vi "Configure Channels.vi"(8 "error in":errorcluster, 11 "DI Cont CFG in":refnum<class "DI DAQmx Cont CFG.lvclass">) -> (0 "error out":errorcluster, 3 "DI Cont CFG out":refnum<class "DI DAQmx Cont CFG.lvclass">)   [LabVIEW 2024, in "DI DAQmx Cont CFG.lvclass"]
uses:
  DI DAQmx Cont CFG.lvclass
  DI DAQmx Cont CFG.lvclass/DI DAQmx Cont CFG.ctl
  DAQmx Base CFG/DAQmx Base CFG.lvclass/DAQmx Base CFG.ctl
  Configurations/CFG Base/CFG Base.lvclass/CFG Base.ctl
  554e4c80-a6e4-4458-875d-47822cf13ff0.vi
  554e4c80-a6e4-4458-875d-47822cf13ff0.vi/a4169a97-72fc-4003-a778-603cf20cafa0.vi
  <vilib>/JDP Science/JSONtext/Find Item.vi
  <vilib>/JDP Science/JSONtext/Next JSON Value.vi
  <vilib>/JDP Science/JSONtext/String Subset.vi
  <vilib>/JDP Science/JSONtext/Parsing/Advance past next JSON Value (inlined COPY).vi
  <vilib>/JDP Science/JSONtext/Parsing/Advance past whitespace.vi
  <vilib>/JDP Science/JSONtext/Parsing/Advance past String.vi
  <vilib>/JDP Science/JSONtext/Parsing/Advance past Number.vi
  <vilib>/JDP Science/JSONtext/Parsing/Advance past Line Ending.vi
  <vilib>/JDP Science/JSONtext/Parsing/Parse Full Path or Item Name.vi
  <vilib>/JDP Science/JSONtext/Parsing/Advance past Array.vi
  <vilib>/JDP Science/JSONtext/Parsing/Advance past Object.vi
  <vilib>/JDP Science/JSONtext/support/Error Cluster From Code.vi
  <vilib>/JDP Science/JSONtext/Offset/Find Item Locations by Path.vi
  <vilib>/JDP Science/JSONtext/JSON text to Variant.vi
  <vilib>/Utility/error.llb/Error Cluster From Error Code.vi
  <vilib>/DAQmx/create/channels.llb/DAQmx Create Channel (DI-Digital Input).vi
  <vilib>/JDP Science/JSONtext/LVClass Serializer/JSONtext LVClass Serializer.lvclass
  Configurations/CFG Base/CFG Base.lvclass
  DAQmx Base CFG/DAQmx Base CFG.lvclass
  Buffers/Buffer Lossless Digital/Buffer Lossless Digital.lvclass
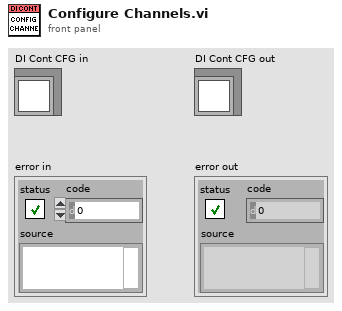
[diagram p1: front panel]
types:
  T1 = cluster{"Name":string, "Enabled":bool, "Line Grouping":string}[]
  T2 = enum16{"one channel for each line", "one channel for all lines"}
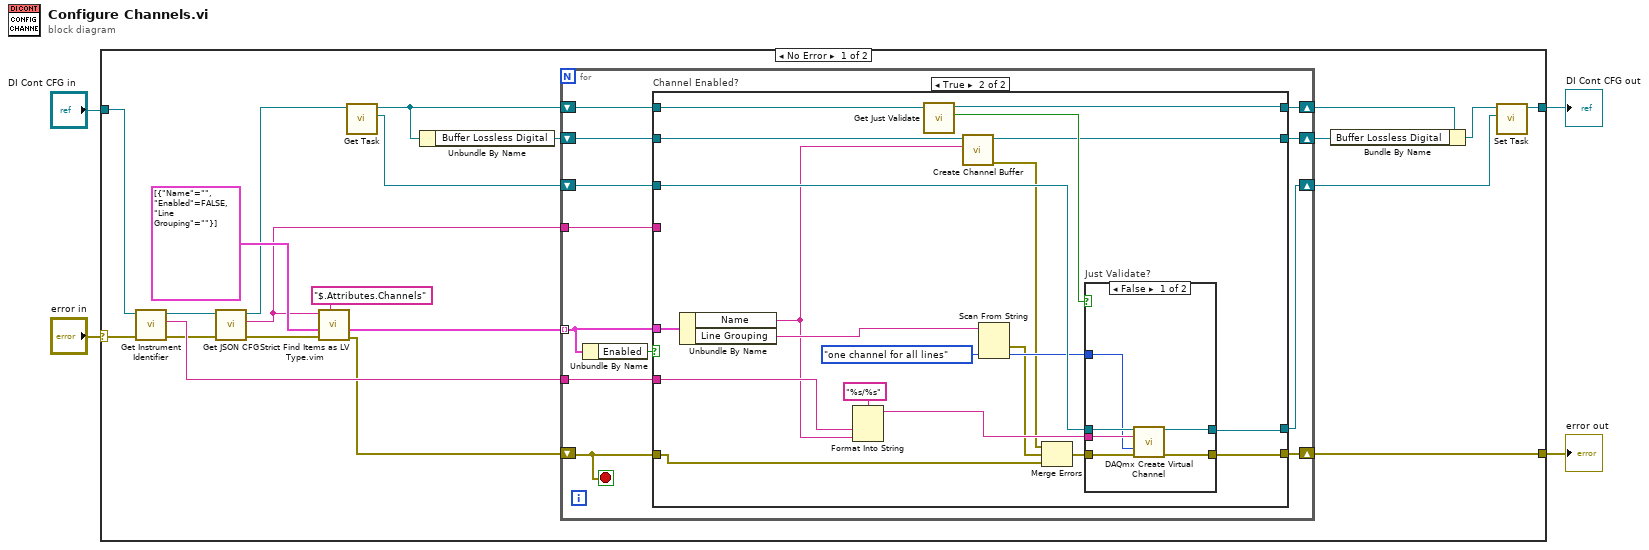
[diagram p0: block diagram]
diagram:
  n1 = case shown="No Error" "error in" {
    selector: "error in" -> [w11 w68]
    tunnel: "DI Cont CFG in" -> [w15 w69]
    tunnel: [w19 w68] -> w4
    tunnel: [w13 w69] -> w2
    frame No Error {
      n2 = call "Get Instrument Identifier.vi"("CFG Base in"=w15) -> ("Instrument Identifier"=w20:string, "CFG Base out"=w21:refnum<class "DI DAQmx Cont CFG.lvclass">)  [unwired: 9 in]
      n3 = call "Get JSON CFG.vi"("CFG Base in"=w21) -> ("<JSON>CFG"=w18:string, "CFG Base out"=w10:refnum<class "DI DAQmx Cont CFG.lvclass">)  [unwired: 9 in]
      n4 = call "Strict Find Items as LV Type.vim"("$Path or Item Name"="$.Attributes.Channels", "error in"=w11, "Data Type and Default Value"=T1 [{"Name"="", "Enabled"=FALSE, "Line Grouping"=""}], "<JSON>"=w18) -> ("error out"=w14:errorcluster, "Data out"=w16:T1)  [unwired: 5 in, 1 out]
      n5 = call "Get Task.vi"("DAQmx Base CFG in"=w10) -> ("Task"=w17:refnum<k21>, "DAQmx Base CFG out"=w9:refnum<class "DI DAQmx Cont CFG.lvclass">)  [unwired: 9 in]
      n6 = Unbundle By Name(w9) -> ("Buffer Lossless Digital"=w8:refnum<class "Buffer Lossless Digital.lvclass">)
      n7 = for {
        tunnel: w16 -> [w32] mode=indexing
        shift-right: [w35] -> w19
        shift-left: w14 -> [w34]
        tunnel: w20 -> [w33]
        tunnel: w18 -> [w31]
        shift-right: [w29] -> w7
        shift-left: w9 -> [w28]
        shift-right: [w26] -> w12
        shift-left: w17 -> [w30]
        shift-right: [w24] -> w5
        shift-left: w8 -> [w25]
        stop <- w34 stop-if-true
        n8 = Unbundle By Name(w32) -> ("Enabled"=w27:bool)
        n9 = case "Channel Enabled?" shown="True" w27 {
          tunnel: [w39 w58] -> w35
          tunnel: w34 -> [w39 w42]
          tunnel: w33 -> [_ w53]
          tunnel: w32 -> [_ w59]
          tunnel: [w38 w40] -> w29
          tunnel: w31 -> [_ _]
          tunnel: w30 -> [w37 w57]
          tunnel: w28 -> [w38 w56]
          tunnel: [w37 w47] -> w26
          tunnel: w25 -> [w36 w46]
          tunnel: [w36 w41] -> w24
          frame False {
          }
          frame True {
            n10 = Unbundle By Name(w59) -> ("Name"=w45:string, "Line Grouping"=w50:string)
            n11 = Format Into String(format string="%s/%s", w53, w45) -> (resulting string=w52:string)  [unwired: 2 in, 1 out]
            n12 = call "Get Just Validate.vi"("CFG Base in"=w56) -> ("Just Validate"=w55:bool, "CFG Base out"=w40:refnum<class "DI DAQmx Cont CFG.lvclass">)  [unwired: 9 in]
            n13 = call "Create Channel Buffer.vi"("Channel"=w45, "Buffer Lossless Dig in"=w46) -> ("error out"=w44:errorcluster, "Buffer Lossless Dig out"=w41:refnum<class "Buffer Lossless Digital.lvclass">)  [unwired: 8 in]
            n14 = Scan From String(input string=w50, default 1=T2."one channel for all lines" ("Line Grouping")) -> (error out=w43:errorcluster, output 1=w49:T2)  [unwired: 3 in, 2 out]
            n15 = Merge Errors(w44, w43, w42) -> (w51:errorcluster)
            n16 = case "Just Validate?" shown="False" w55 {
              tunnel: w51 -> [w65 w67]
              tunnel: w52 -> [w61 _]
              tunnel: w57 -> [w64 w66]
              tunnel: [w63 w67] -> w58
              tunnel: w49 -> [w60 _]
              tunnel: [w62 w66] -> w47
              frame False {
                n17 = call-poly <vilib>:"DAQmx Create Virtual Channel.vi"("task in"=w64, "lines"=w61, "line grouping"=w60, "error in"=w65) -> ("task out"=w62:refnum<k21>, "error out"=w63:errorcluster)  [unwired: 10 in]
              }
              frame True {
              }
            }
          }
        }
      }
      n18 = Bundle By Name(cluster=w7, "Buffer Lossless Digital"=w5) -> (w6:refnum<class "DI DAQmx Cont CFG.lvclass">)
      n19 = call "Set Task.vi"("Task"=w12, "DAQmx Base CFG in"=w6) -> ("DAQmx Base CFG out"=w13:refnum<class "DI DAQmx Cont CFG.lvclass">)  [unwired: 9 in]
    }
    frame Error {
    }
  }
  "error out" <- w4
  "DI Cont CFG out" <- w2
